vi "FVI_Trajectiore_Swerve4vitesse.vi"(0 "Vx":dbl, 1 "Gain":dbl=1.0, 5 "Vy":dbl, 7 "Omega":dbl, 12 "Longueur":dbl, 13 "Largeur":dbl) -> (4 "SwerveDrive":T1)   [LabVIEW 2018]
uses:
  SwerveDrive.ctl
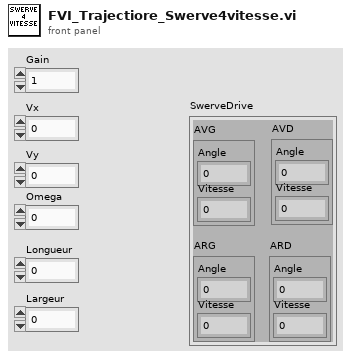
[diagram p1: front panel]
types:
  T1 = typedef "SwerveDrive.ctl" = cluster{"AVD":cluster{"Angle":dbl, "Vitesse":dbl}, "AVG":cluster{"Angle":dbl, "Vitesse":dbl}, "ARG":cluster{"Angle":dbl, "Vitesse":dbl}, "ARD":cluster{"Angle":dbl, "Vitesse":dbl}}
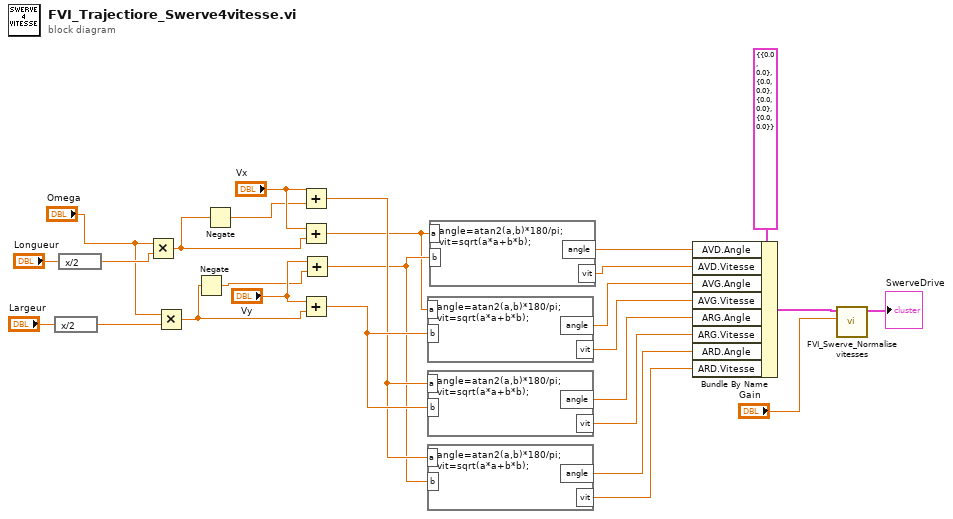
[diagram p0: block diagram]
diagram:
  n1 = expression code="x/2"("Largeur") -> (w5:dbl)
  n2 = expression code="x/2"("Longueur") -> (w25:dbl)
  n3 = Multiply(x="Omega", y=w25) -> (x*y=w21:dbl)
  n4 = Multiply(x="Omega", y=w5) -> (x*y=w2:dbl)
  n5 = Negate(x=w2) -> (-x=w3:dbl)
  n6 = Negate(x=w21) -> (-x=w22:dbl)
  n7 = Add(x="Vx", y=w22) -> (x+y=w17:dbl)
  n8 = Add(x="Vx", y=w21) -> (x+y=w7:dbl)
  n9 = Add(x="Vy", y=w2) -> (x+y=w18:dbl)
  n10 = Add(x="Vy", y=w3) -> (x+y=w16:dbl)
  n11 = formula code="angle=atan2(a,b)*180/pi;\nvit=sqrt(a*a+b*b);"("a"=w7, "b"=w18) -> ("angle"=w15:dbl, "vit"=w14:dbl)
  n12 = formula code="angle=atan2(a,b)*180/pi;\nvit=sqrt(a*a+b*b);"("a"=w17, "b"=w18) -> ("angle"=w13:dbl, "vit"=w12:dbl)
  n13 = formula code="angle=atan2(a,b)*180/pi;\nvit=sqrt(a*a+b*b);"("a"=w17, "b"=w16) -> ("angle"=w11:dbl, "vit"=w10:dbl)
  n14 = formula code="angle=atan2(a,b)*180/pi;\nvit=sqrt(a*a+b*b);"("a"=w7, "b"=w16) -> ("angle"=w20:dbl, "vit"=w19:dbl)
  n15 = Bundle By Name(cluster=T1 {"AVD"={"Angle"=0.0, "Vitesse"=0.0}, "AVG"={"Angle"=0.0, "Vitesse"=0.0}, "ARG"={"Angle"=0.0, "Vitesse"=0.0}, "ARD"={"Angle"=0.0, "Vitesse"=0.0}} ("SwerveDrive"), "AVD.Angle"=w20, "AVD.Vitesse"=w19, "AVG.Angle"=w15, "AVG.Vitesse"=w14, "ARG.Angle"=w13, "ARG.Vitesse"=w12, "ARD.Angle"=w11, "ARD.Vitesse"=w10) -> (w9:T1)
  n16 = call "FVI_Swerve_Normalise vitesses.vi"("Gain"="Gain", "SwerveDrive in"=w9) -> ("SwerveDrive out"=→"SwerveDrive":T1)  [unwired: 9 in]
